vi "Load Waveform Chart History - multiple plots.vi"(8 "error in (no error)":errorcluster, 10 "Plot GUI label":string, 11 "Father of all uServices in":refnum<class "Father of all uServices.lvclass">) -> (0 "error out":errorcluster, 2 "History Data - multiple plots":waveform(dbl)[][](array[waveform]), 3 "Father of all uServices out":refnum<class "Father of all uServices.lvclass">)   [LabVIEW 2026, in "TALOS.lvlib" / "Father of all uServices.lvlib" / "Father of all uServices.lvclass"]
uses:
  Father of all uServices.lvclass
  Children Methods/Waveform Chart Class Reference Strict - multiple plots.ctl
  Ancestor/Ancestor/Ancestor.lvclass/Ancestor.ctl
  Support VIs/Generate Error.vi
  FGV/Error Memory/Get Error Description.vi
  Support VIs/Get PC name.vi
  Ancestor/Ancestor/Read ID.vi
  Support VIs/Get Class Name.vi
  FGV/Error Memory/Error Memory Core.vi
  <vilib>/AdvancedString/Delimited String to 1D String Array.vi
  <vilib>/AdvancedString/Delimited String to 1D String Array (string).vi
  Support VIs/Circus Root Path.vi
  FGV/Error Memory/Error Crt Lvl checker.vi
  FGV/Error Memory/Error Memory Core.vi/40c8088d-b597-4017-91af-faa98e00292e.vi
  FGV/Error Memory/Error Memory Core.vi/d4a3ab98-063c-4e44-b43d-fbdcfe6c2be2.vi
  <vilib>/Utility/file.llb/Read Delimited Spreadsheet (DBL).vi
  Support VIs/Global Memory.vi
  <vilib>/Utility/LVClass/Get LV Class Name.vi
  Support VIs/Is in Packed Library.vi
  Support VIs/TALOS Root path.vi
  Support VIs/Read CSV worksheet.vi
  Support VIs/Global Constants.vi
  <vilib>/Utility/error.llb/General Error Handler.vi
  Ancestor/Ancestor/Ancestor.lvclass
  <vilib>/Comparison/Equal/Equal Functor/Equal Functor.lvclass
  TALOS.lvlib
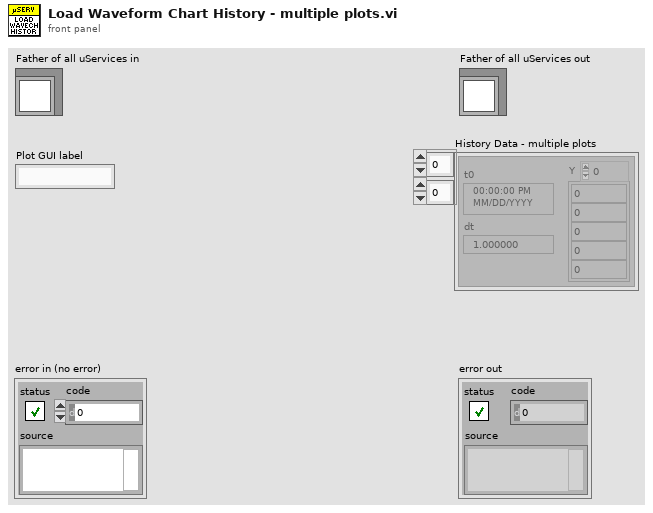
[diagram p1: front panel]
types:
  T1 = typedef "TALOS.lvlib/Father of all uServices.lvlib/Father of all uServices.lvclass/Waveform Chart Class Reference Strict - multiple plots.ctl" = refnum<vi>
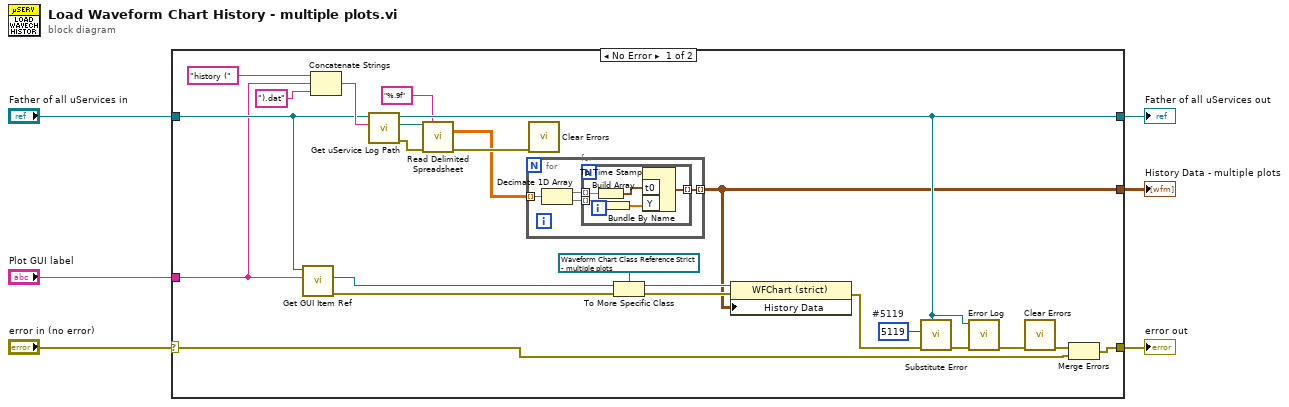
[diagram p0: block diagram]
diagram:
  n1 = case shown="No Error" "error in (no error)" {
    selector: "error in (no error)" -> [w7 w41]
    tunnel: [w8 w41] -> w5
    tunnel: [w24 w40] -> w3
    tunnel: "Father of all uServices in" -> [w15 w40]
    tunnel: "Plot GUI label" -> [w14 _]
    tunnel: [w9 _] -> w1
    frame No Error {
      w27 = 5119  # #5119
      n2 = call "Get GUI Item Ref.vi"("FP Item Name"=w14, "uService Template in"=w15) -> ("error out"=w12:errorcluster, "Ctl Refnum"=w13:refnum<vi>)  [unwired: 7 in, 1 out]
      n3 = Concatenate Strings("history (" ("string"), w14, ").dat" ("string")) -> (w28:string)
      n4 = call "Get uService Log Path.vi"("Log File Suffix"=w28, "Father of all uServices in"=w15) -> ("error out"=w18:errorcluster, "Log File Path"=w19:path, "Father of all uServices out"=w24:refnum<class "Father of all uServices.lvclass">)  [unwired: 7 in]
      n5 = call-poly <vilib>:"Read Delimited Spreadsheet.vi"("file path (dialog if empty)"=w19, "format (%.3f)"="%.9f", "error in (no error)"=w18) -> ("all rows"=w10:dbl[][], "error out"=w11:errorcluster)  [unwired: 7 in, 4 out]
      n6 = for {
        tunnel: w10 -> [w34] mode=indexing
        tunnel: [w31] -> w9 mode=indexing
        n7 = Decimate 1D Array(w34) -> (w33:dbl[], w32:dbl[])
        n8 = for {
          tunnel: w33 -> [w39] mode=indexing
          tunnel: w32 -> [w38] mode=indexing
          tunnel: [w35] -> w31 mode=indexing
          n9 = To Time Stamp(1:w39) -> (0:w37:timestamp)
          n10 = Build Array(w38) -> (w36:dbl[])
          n11 = Bundle By Name("t0"=w37, "Y"=w36) -> (w35:waveform(dbl))  [unwired: 1 in]
        }
      }
      n12 = call <vilib>:"Clear Errors.vi"("error in (no error)"=w11) -> ()  [unwired: 5 in, 2 out]
      n13 = To More Specific Class(target class=T1 refnum ("Waveform Chart - multiplot"), reference=w13, error in=w12) -> (specific class reference=w21:T1, error out=w20:errorcluster)
      n14 = property class="WFChart (strict)"(reference=w21, error in=w20, "History Data"=w9) -> (error out=w26:errorcluster)  [unwired: 1 out]
      n15 = call "Substitute Error.vi"("LabVIEW Object"=w24, "error in (no error)"=w26, "Error Code"=w27) -> ("error out"=w25:errorcluster)  [unwired: 8 in]
      n16 = call "Error Log.vi"("error in (no error)"=w25, "Object in"=w24) -> ("error out"=w23:errorcluster)  [unwired: 9 in]
      n17 = call <vilib>:"Clear Errors.vi"("error in (no error)"=w23) -> ("error out"=w22:errorcluster)  [unwired: 5 in, 1 out]
      n18 = Merge Errors(w22, w7) -> (w8:errorcluster)
    }
    frame Error {
    }
  }
  "error out" <- w5
  "Father of all uServices out" <- w3
  "History Data - multiple plots" <- w1
